vi "Main.vi"(6 "Folder names":string[](array[string])=["StaARx#[PLC]StaATesterRxSignals", "StaATx#[PLC]StaATesterTxSignals"], 8 "error in":errorcluster, 9 "Sequence Context In":refnum<k7>, 10 "OPC UA refnum":T1, 11 "TestExec In":refnum<class "TestExec.lvclass">) -> (0 "error out":errorcluster, 3 "TestExec Out":refnum<class "TestExec.lvclass">)   [LabVIEW 2019, in "OPC UA.lvlib" / "TestExec.lvclass"]
uses:
  TestExec.lvclass
  TestExec.lvclass/TestExec.ctl
  Methods/Cylinder Display.vi
  <vilib>/addons/TestStand/_TSUtility.llb/TestStand - Get Property Value (Number {Signed 32-bit Integer}).vi
  OPC UA/OPC UA.lvclass
  <vilib>/OPCUA/controls/OPC UA Client Refnum.ctl
panel:
  in  "Terminate":bool
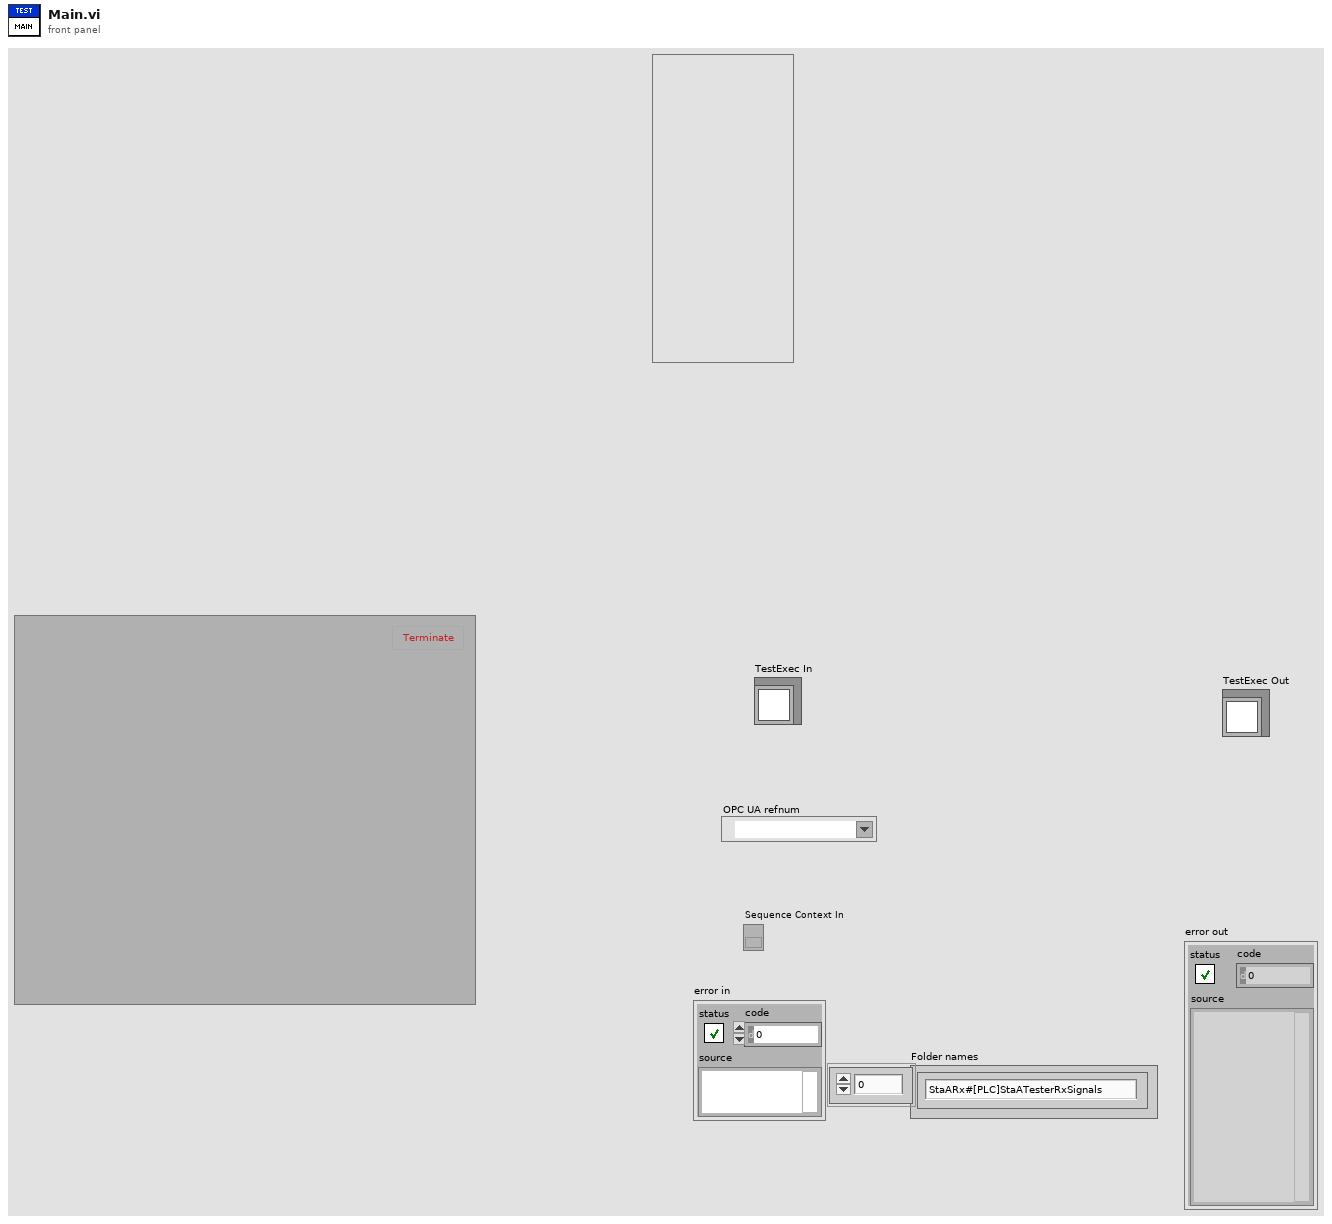
[diagram p1: front panel]
types:
  T1 = typedef "OPC UA Client Refnum.ctl" = refnum<k21>
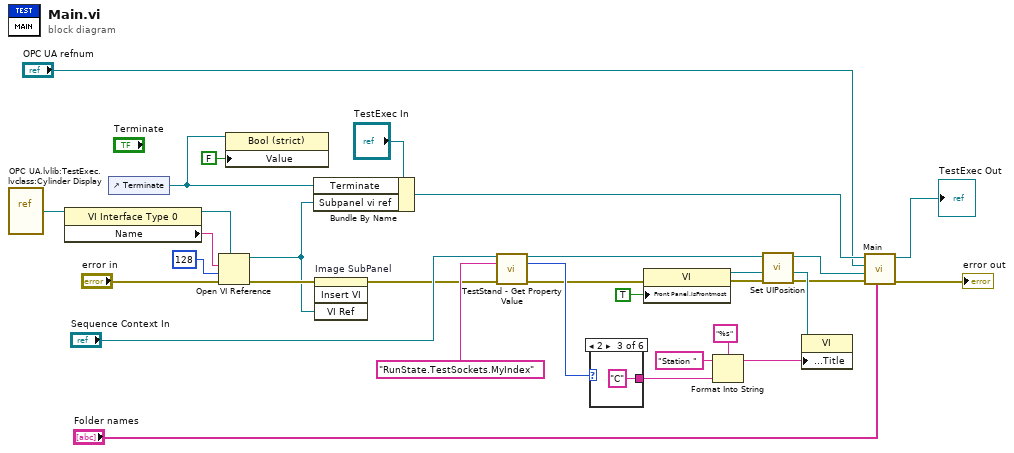
[diagram p0: block diagram]
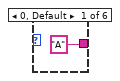
[diagram p2: hidden frame]
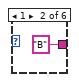
[diagram p3: hidden frame]
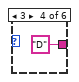
[diagram p4: hidden frame]
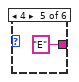
[diagram p5: hidden frame]
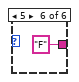
[diagram p6: hidden frame]
diagram:
  n1 = vi-ref "OPC UA.lvlib:TestExec.lvclass:Cylinder Display.vi"() -> (w26:refnum<vi>)
  n2 = property on="Property Node" class="VI Interface Type 0"(reference=w26) -> (reference out=w28:refnum<vi>, "Name"=w27:string)  [unwired: 1 in, 1 out]
  n3 = control-ref of="Terminate"() -> (w3:refnum<vi>)
  n4 = Open VI Reference(type specifier VI Refnum (for type only)=w28, vi path=w27, options=128, error in (no error)="error in") -> (vi reference=w22:refnum<vi>, error out=w23:errorcluster)  [unwired: 2 in]
  n5 = property class="Bool (strict)"(reference=w3, "Value"=FALSE) -> ()  [unwired: 1 in, 2 out]
  n6 = Bundle By Name(cluster="TestExec In", "Terminate"=w3, "Subpanel vi ref"=w22) -> (w20:refnum<class "TestExec.lvclass">)
  n7 = invoke on="Image SubPanel" class="SubPnl" method="Insert VI"(error in=w23, "VI Ref"=w22) -> (error out=w4:errorcluster)  [unwired: 2 in, 3 out]
  n8 = call-poly <vilib>:"TestStand - Get Property Value.vi"("Sequence Context In"="Sequence Context In", "Lookup String"="RunState.TestSockets.MyIndex", "error in (no error)"=w4) -> ("Sequence Context Out"=w8:refnum<k7>, "Value"=w11:i32, "error out"=w5:errorcluster)  [unwired: 10 in]
  n9 = case shown="2" w11 {
    tunnel: ["A" ("format string") "B" ("format string") "C" ("format string") "D" ("format string") "E" ("format string") "F" ("format string")] -> w16
    frame 0, Default {
    }
    frame 1 {
    }
    frame 2 {
    }
    frame 3 {
    }
    frame 4 {
    }
    frame 5 {
    }
  }
  n10 = property class="VI"(error in=w5, "Front Panel.IsFrontmost"=TRUE ("Front Panel Window:Is Frontmost")) -> (reference out=w17:refnum<vi>, error out=w18:errorcluster)  [unwired: 1 in]
  n11 = Format Into String(format string="%s", initial string="Station ", w16) -> (resulting string=w10:string)  [unwired: 1 in, 1 out]
  n12 = call "Set UIPosition.vi"("error in"=w18, "VI Ref"=w17, "Sequence Context In"=w8) -> ("error out"=w6:errorcluster, "reference out"=w9:refnum<vi>, "Sequence Context Out"=w7:refnum<k7>)  [unwired: 6 in]
  n13 = property class="VI"(reference=w9, "Front Panel.Title"=w10) -> ()  [unwired: 1 in, 2 out]
  n14 = call-parent "Main.vi"("Folder names"="Folder names", "error in"=w6, "Sequence Context"=w7, "OPC UA refnum"="OPC UA refnum", "OPC UA In"=w20) -> ("error out"=→"error out":errorcluster, "OPC UA Out"=→"TestExec Out":refnum<class "TestExec.lvclass">)  [unwired: 5 in]
